vi "test_Create Data Channel_single channel comparison.vi"(8 "error in (no error)":errorcluster, 11 "TestCase in":refnum<class "Instrument Addon Scripting API Channels Unit Tests.lvclass">) -> (0 "error out":errorcluster, 3 "TestCase out":refnum<class "Instrument Addon Scripting API Channels Unit Tests.lvclass">)   [LabVIEW 2019, in "Instrument Addon Scripting API Channels Unit Tests.lvclass"]
uses:
  Instrument Addon Scripting API Channels Unit Tests.lvclass
  APIs/Scripting API/TypeDefs/Single Channel Comparison Settings.ctl
  Addon/Addon Shared/Types/Protocol Data Type.ctl
  Addon/Addon Shared/Types/Data Channel Type.ctl
  Instrument Addon Scripting API Channels Unit Tests.lvclass/Instrument Addon Scripting API Channels Unit Tests.ctl
  Addon/Addon Shared/SubVIs/Constants.vi
  <vilib>/NI/NI VeriStand Advanced SysDef API/_SubVIs/SysDef.Search.GUID.vi
  <vilib>/NI/NI VeriStand Advanced SysDef API/_SubVIs/SysDef.Search.GUIDs.vi
  APIs/Scripting API/Channels/Create Data Channel - Single Channel - Comparison.vi
  <vilib>/NI VeriStand/Custom Device API/Get Item Property (U16).vi
  <vilib>/NI VeriStand/Custom Device API/Get Item Property (String).vi
  <vilib>/addons/_JKI Toolkits/VI Tester/TestCase.llb/TestCase.lvclass
  Instrument Addon Scripting API Test Assets/Instrument Addon Scripting API Test Assets.lvclass
  <vilib>/NI/NI VeriStand Advanced SysDef API/SysDef API/Advanced System Definition.lvlib
  Addon/Addon Shared/Instrument Addon Shared.lvlib
  <vilib>/NI VeriStand/Custom Device API/Custom Device API.lvlib
  APIs/Scripting API/Instrument Addon Scripting API.lvlib
  C:/Program Files (x86)/National Instruments/LabVIEW 2019/vi.lib/addons/_JKI Toolkits/VI Tester/TestCase.llb/TestCase.lvclass
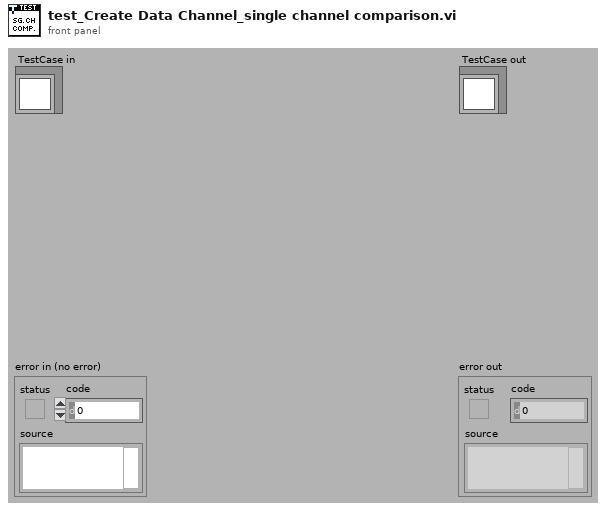
[diagram p1: front panel]
types:
  T1 = typedef "Instrument Addon Scripting API.lvlib/Single Channel Comparison Settings.ctl" = cluster{"Expected String(case sensitive)":string, "Default Value":dbl, "Units":string}
  T2 = typedef "Instrument Addon Shared.lvlib/Data Channel Type.ctl" = enum16{"Format", "Comparison", "Type Cast", "Enumerated List"}
  T3 = typedef "Instrument Addon Shared.lvlib/Protocol Data Type.ctl" = enum16{"Single Channel", "Array"}
  T4 = typedef "Custom Device API.lvlib/Custom Device Item Ref.ctl" = u64
  T5 = typedef "Custom Device API.lvlib/Custom Device Channel.ctl" = cluster{"Type":T6, "Units":string, "Default Value":dbl, "Faultable":bool, "Scalable":bool}
  T6 = typedef "Custom Device API.lvlib/Custom Device Channel Type.ctl" = enum16{"Input", "Output"}
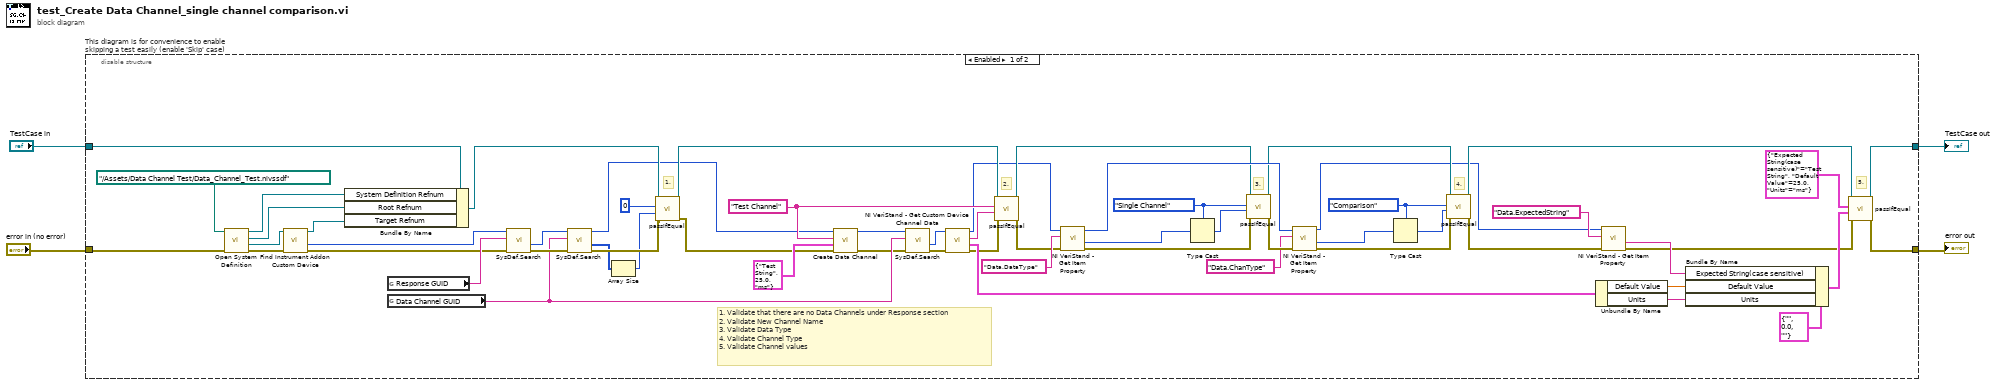
[diagram p0: block diagram]
diagram:
  n1 = disable-structure "This diagram is for convenience to enable skipping a test easily (enable 'Skip' case)" shown="Enabled" {
    disable-tunnel: "TestCase in" -> [w32 w68]
    disable-tunnel: [w64 w66] -> w1
    disable-tunnel: [w63 w67] -> w3
    disable-tunnel: "error in (no error)" -> [w60 w65]
    frame Enabled {
      w16 = Data_Channel_Type."Comparison" ("Channel Type")
      w21 = Protocol_Data_Type."Single Channel" ("Data Type")
      w43 = "Test Channel" ("Name")
      # "1. Validate that there are no Data Channels under Response section\n2. Validate New Channel Name\n3. Validate Data Type\n4. Validate Channel Type\n5. Validate Channel values"
      # "4."
      # "3."
      # "5."
      # "2."
      # "1."
      n2 = call "Open System Definition.vi"("error in (no error)"=w60, "System Definition File"=path "../Assets/Data Channel Test/Data_Channel_Test.nivssdf") -> ("error out"=w62:errorcluster, "Target Refnum"=w30:refnum<k24>, "Root Refnum"=w34:refnum<k24>, "System Definition Refnum"=w35:refnum<k24>)  [unwired: 6 in]
      n3 = call "Find Instrument Addon Custom Device.vi"("error in"=w62, "target in"=w30) -> ("error out"=w29:errorcluster, "NodeID"=w59:u64, "target out"=w33:refnum<k24>)  [unwired: 7 in]
      n4 = Bundle By Name(cluster=w32, "System Definition Refnum"=w35, "Root Refnum"=w34, "Target Refnum"=w33) -> (w31:refnum<class "Instrument Addon Scripting API Channels Unit Tests.lvclass">)
      n5 = global read "Constants.vi" "Response GUID"() -> (w58:string)
      n6 = global read "Constants.vi" "Data Channel GUID"() -> (w55:string)
      n7 = call-poly <vilib>:"SysDef.Search.vi"("error in (no error)"=w29, "GUID"=w58, "nodeID"=w59) -> ("error out"=w56:errorcluster, "Value out"=w57:u64)  [unwired: 5 in, 2 out]
      n8 = call-poly <vilib>:"SysDef.Search.vi"("error in (no error)"=w56, "GUID"=w55, "nodeID"=w57) -> ("error out"=w47:errorcluster, "Values Out"=w46:u64[], "nodeID out"=w5:u64)  [unwired: 5 in, 1 out]
      n9 = Array Size(array=w46) -> (size(s)=w45:i32)
      n10 = call-dynamic "passIfEqual.vi"("error in (no error)"=w47, "y"=w45, "x"=0 ("size(s)"), "TestCase in"=w31) -> ("error out"=w28:errorcluster, "TestCase out"=w26:refnum<class "Instrument Addon Scripting API Channels Unit Tests.lvclass">)  [unwired: 6 in]
      n11 = call-poly "Create Data Channel.vi"("error in (no error)"=w28, "settings"=T1 {"Expected String(case sensitive)"="Test String", "Default Value"=25.0, "Units"="ms"} ("Settings"), "channel name"=w43, "response refnum in"=w5) -> ("error out"=w41:errorcluster, "response refnum out"=w42:T4)  [unwired: 5 in, 1 out]
      n12 = call-poly <vilib>:"SysDef.Search.vi"("error in (no error)"=w41, "GUID"=w55, "nodeID"=w42) -> ("error out"=w54:errorcluster, "Value out"=w40:u64)  [unwired: 5 in, 2 out]
      n13 = call <vilib>:"NI VeriStand - Get Custom Device Channel Data.vi"("error in (no error)"=w54, "Channel Ref in"=w40) -> ("error out"=w27:errorcluster, "Channel"=w53:T5, "Channel Name"=w49:string, "Channel Ref out"=w10:T4)  [unwired: 4 in, 2 out]
      n14 = call-dynamic "passIfEqual.vi"("error in (no error)"=w27, "y"=w49, "x"=w43, "TestCase in"=w26) -> ("error out"=w12:errorcluster, "TestCase out"=w11:refnum<class "Instrument Addon Scripting API Channels Unit Tests.lvclass">)  [unwired: 6 in]
      n15 = call-poly <vilib>:"NI VeriStand - Get Item Property.vi"("error in (no error)"=w12, "Property Name"="Data.DataType", "Item Ref in"=w10) -> ("error out"=w24:errorcluster, "Value"=w23:u16, "Item Ref out"=w15:T4)  [unwired: 5 in, 1 out]
      n16 = Type Cast(type=w21, x=w23) -> (*(type *) &x=w22:T3)
      n17 = call-dynamic "passIfEqual.vi"("error in (no error)"=w24, "y"=w22, "x"=w21, "TestCase in"=w11) -> ("error out"=w20:errorcluster, "TestCase out"=w13:refnum<class "Instrument Addon Scripting API Channels Unit Tests.lvclass">)  [unwired: 6 in]
      n18 = call-poly <vilib>:"NI VeriStand - Get Item Property.vi"("error in (no error)"=w20, "Property Name"="Data.ChanType", "Item Ref in"=w15) -> ("error out"=w19:errorcluster, "Value"=w18:u16, "Item Ref out"=w6:T4)  [unwired: 5 in, 1 out]
      n19 = Type Cast(type=w16, x=w18) -> (*(type *) &x=w17:T2)
      n20 = call-dynamic "passIfEqual.vi"("error in (no error)"=w19, "y"=w17, "x"=w16, "TestCase in"=w13) -> ("error out"=w9:errorcluster, "TestCase out"=w8:refnum<class "Instrument Addon Scripting API Channels Unit Tests.lvclass">)  [unwired: 6 in]
      n21 = Unbundle By Name(w53) -> ("Default Value"=w52:dbl, "Units"=w51:string)
      n22 = call-poly <vilib>:"NI VeriStand - Get Item Property.vi"("error in (no error)"=w9, "Property Name"="Data.ExpectedString", "Item Ref in"=w6) -> ("error out"=w7:errorcluster, "Value"=w37:string)  [unwired: 5 in, 2 out]
      n23 = Bundle By Name(cluster=T1 {"Expected String(case sensitive)"="", "Default Value"=0.0, "Units"=""} ("Settings"), "Expected String(case sensitive)"=w37, "Default Value"=w52, "Units"=w51) -> (w48:T1)
      n24 = call-dynamic "passIfEqual.vi"("error in (no error)"=w7, "y"=w48, "x"=T1 {"Expected String(case sensitive)"="Test String", "Default Value"=25.0, "Units"="ms"} ("Settings"), "TestCase in"=w8) -> ("error out"=w63:errorcluster, "TestCase out"=w64:refnum<class "Instrument Addon Scripting API Channels Unit Tests.lvclass">)  [unwired: 6 in]
    }
    frame Disabled {
      # "skip test result while test is under development"
      n25 = call <vilib>:"skip.vi"("error in (no error)"=w65, "TestCase in"=w68) -> ("error out"=w67:errorcluster, "TestCase out"=w66:refnum<class "Instrument Addon Scripting API Channels Unit Tests.lvclass">)  [unwired: 8 in]
    }
  }
  "error out" <- w3
  "TestCase out" <- w1
